vi "20220302-main.vi"() -> ()   [LabVIEW 2019]
uses:
  <vilib>/myRIO/Instrument Drivers/Utilities/Utilities.lvlib
  52/sub/servo state.ctl
  52/sub/state.ctl
  52/sub/route_name.ctl
  52/main data.ctl
  52/sub/vision/vision_board_ctl.ctl
  52/sub/block box.ctl
  52/sub/align position.ctl
  <vilib>/myRIO/Common/Instrument Driver Framework/myRIO v1.0/DIO/typedefs/DIO Channels Enum.ctl
  <vilib>/myRIO/Common/Instrument Driver Framework/myRIO v1.0/DIO/typedefs/DIO Channels List.ctl
  <vilib>/myRIO/Common/Instrument Driver Framework/Utilities/typedefs/Generic FPGA Reference.ctl
  <vilib>/myRIO/Common/Instrument Driver Framework/Utilities/typedefs/myRIO v1.0 Reference.ctl
  <vilib>/myRIO/Common/Instrument Driver Framework/Utilities/typedefs/Hardware Version Enum.ctl
  <vilib>/myRIO/Common/Instrument Driver Framework/Utilities/typedefs/myRIO Generic Hardware Reference.ctl
  <vilib>/myRIO/Instrument Drivers/Onboard IO/DIO/typedefs/DIO Reference.ctl
  <vilib>/myRIO/Instrument Drivers/Onboard IO/DIO/DIO.lvlib
  <vilib>/myRIO/Instrument Drivers/Onboard IO/DIO/vis/Write.vi
  <vilib>/userDefined/High Color/nirio_resource_hc.ctl
  <vilib>/myRIO/Common/Instrument Driver Framework/myRIO v1.0/DIO/vis/myRIO v1.1 Open DIO.vi
  <vilib>/myRIO/Instrument Drivers/Onboard IO/DIO/vis/myRIO DIO Open.xnode
  <vilib>/myRIO/Common/Instrument Driver Framework/Utilities/vis/Is FPGA Ref Available.vi
  <vilib>/myRIO/Express VI/Onboard Devices/LED/LED Express VI.xnode
  <vilib>/myRIO/Instrument Drivers/Onboard IO/DIO/vis/Read.vi
  <vilib>/myRIO/Express VI/Onboard Devices/Button/Button Express VI.xnode
  subVI/move control/move and align/move_cluster.ctl
  <vilib>/myRIO/Express VI/Onboard IO/DO/DO Express VI.xnode
panel:
  out "main.ctl":T1
  out "recycle?":bool
  in  "Error In":errorcluster
  out "error out":errorcluster
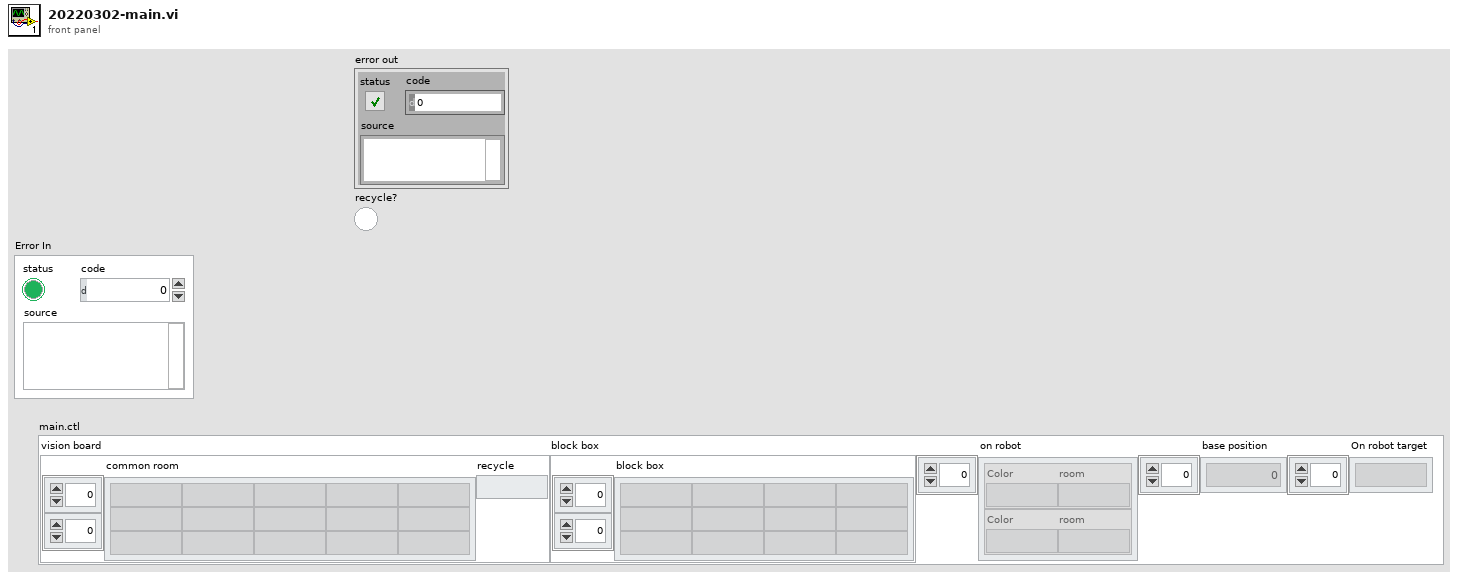
[diagram p1: front panel]
types:
  T1 = typedef "main data.ctl" = cluster{"vision board":T2, "block box":T3, "on robot ":cluster{"Color":string, "room":string}[], "base position":dbl[], "On robot target":string[]}
  T2 = typedef "vision_board_ctl.ctl" = cluster{"common room":string[][], "recycle":string}
  T3 = typedef "block box.ctl" = cluster{"block box":string[][]}
  T4 = typedef "state.ctl" = enum16{"vision", "catch", "recycle", "go home"}
  T5 = typedef "DIO.lvlib/DIO Reference.ctl" = cluster{"myRIO Reference":T6, "DIO Channels List":T10}
  T6 = typedef "myRIO Generic Hardware Reference.ctl" = cluster{"myRIO Model":T7, "myRIO Hardware Reference":T8}
  T7 = typedef "Hardware Version Enum.ctl" = enum16{"Unknown", "myRIO-1900", "myRIO-1950", "roboRIO", "NI ELVIS RIO CM", "ELVIS III"}
  T8 = typedef "myRIO v1.0 Reference.ctl" = cluster{"Generic FPGA Reference":T9, "Allow multiple opens":bool}
  T9 = typedef "Generic FPGA Reference.ctl" = refnum<k20>
  T10 = typedef "DIO Channels List.ctl" = T11[]
  T11 = typedef "DIO Channels Enum.ctl" = enum16{"Not Connected", "C/DIO0", "C/DIO1", "C/DIO2", "C/DIO3", "C/DIO4", "C/DIO5", "C/DIO6", "C/DIO7", "A/DIO0", "A/DIO1", "A/DIO2", "A/DIO3", "A/DIO4", "A/DIO5", "A/DIO6", "A/DIO7", "A/DIO8", "A/DIO9", "A/DIO10", "A/DIO11", "A/DIO12", "A/DIO13", "A/DIO14", "A/DIO15", "A/DIO16", "A/DIO17", "A/DIO18", "A/DIO19", "B/DIO0", "B/DIO1", "B/DIO2", "B/DIO3", "B/DIO4", "B/DIO5", "B/DIO6", "B/DIO7", "B/DIO8", "B/DIO9", "B/DIO10", "B/DIO11", "B/DIO12", "B/DIO13", "B/DIO14", "B/DIO15", "B/DIO16", "B/DIO17", "B/DIO18", "B/DIO19", "LED0", "LED1", "LED2", "LED3", "Button0", "DIO/DIO0", "DIO/DIO1", "DIO/DIO2", "DIO/DIO3", "DIO/DIO4", "DIO/DIO5", "DIO/DIO6", "DIO/DIO7", "DIO/DIO8", "DIO/DIO9", "SPI/CS0", "SPI/CS1", "SPI/CS2", "SPI/CS3", "LED RADIO (Green)", "LED RADIO (Red)", "LED COMM (Green)", "LED COMM (Red)", "LED MODE (Green)", "LED MODE (Red)"}
  T12 = typedef "nirio_resource_hc.ctl" = tag
  T13 = typedef "move_cluster.ctl" = cluster{"X":dbl, "Y":dbl, "degree":dbl, "speed":dbl}
  T14 = typedef "route_name.ctl" = enum16{"S-Vision", "Vision-R1", "Vision-R2", "Vision-R3", "Vision-R4", "Vision-R5", "R1-Vision", "R2-Vision", "R3-Vision", "R4-Vision", "R5-Vision", "Vision-box", "box-recycle", "recycle-box", "box-Vision", "Vision-S", "R2-R3"}
  T15 = typedef "servo state.ctl" = enum16{"catch", "cam-1", "put", "side", "center", "side-2", "put-2"}
  T16 = typedef "align position.ctl" = enum16{"S align", "vision align", "box align", "box to room align"}
  T17 = typedef "position cluster.ctl" = cluster{"X":dbl, "Y":dbl, "Angle":dbl}
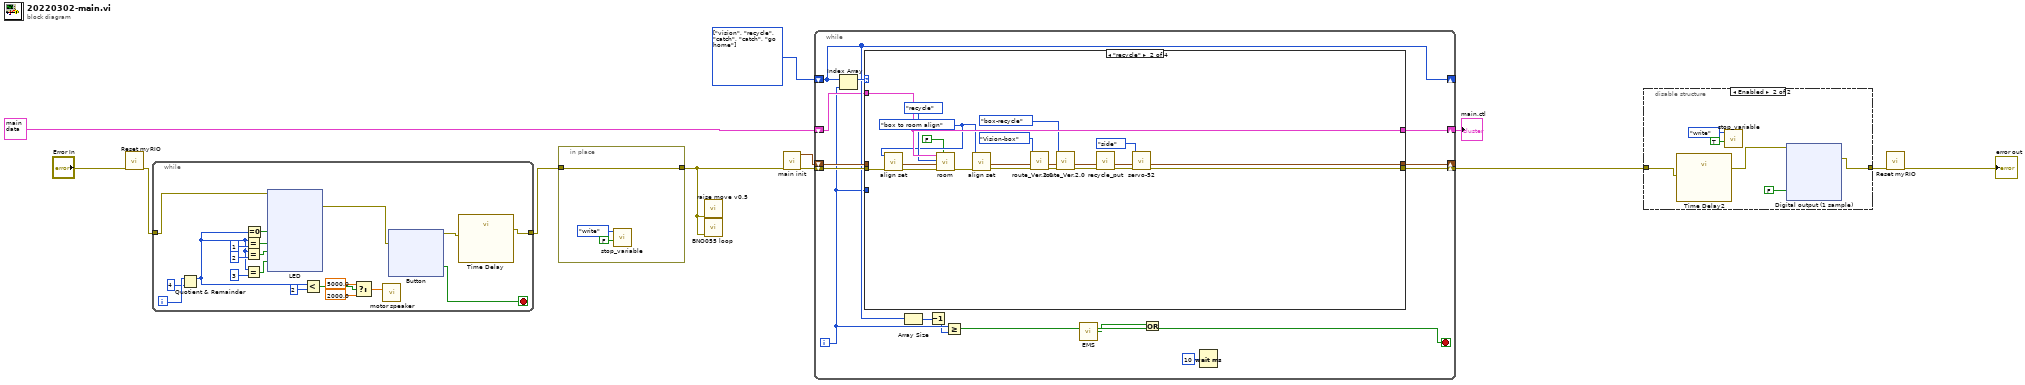
[diagram p0: block diagram]
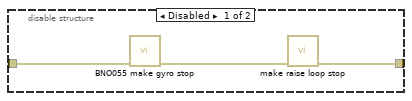
[diagram p2: hidden frame]
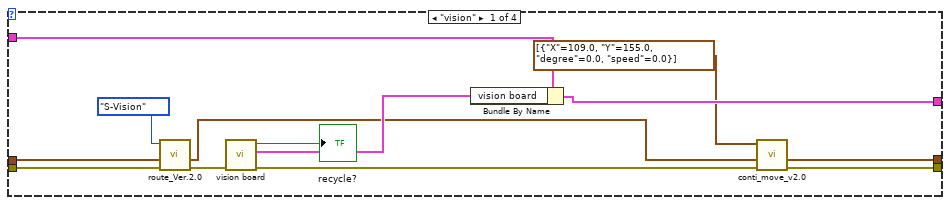
[diagram p3: hidden frame]
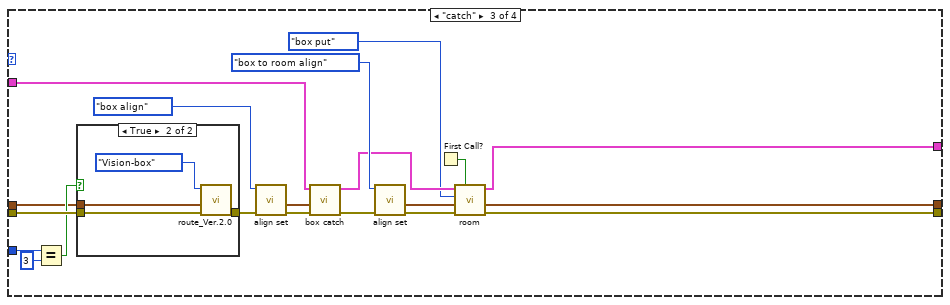
[diagram p4: hidden frame]
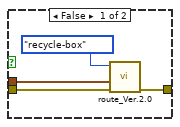
[diagram p5: hidden frame]
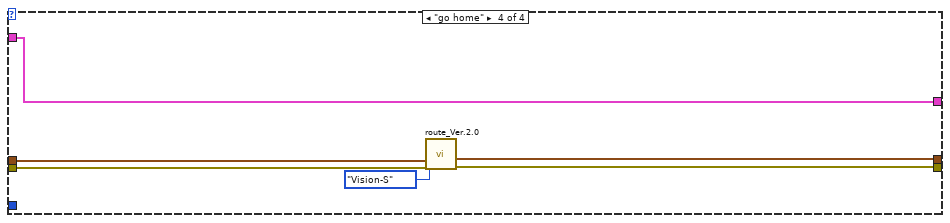
[diagram p6: hidden frame]
diagram:
  w9 = T4[] [enum."vision", enum."recycle", enum."catch", enum."catch", enum."go home"] items=["vision", "catch", "recycle", "go home"] ("Array")
  n1 = call <vilib>:"Reset myRIO.vi"("error in (no error)"="Error In") -> ("error out"=w2:errorcluster)  [unwired: 10 in]
  n2 = while {
    tunnel: w2 -> [w23]
    tunnel: [w20] -> w1
    i -> [w32]
    stop <- w21 stop-if-true
    n3 = Quotient & Remainder(x=w32, y=4) -> (x-y*floor(x/y)=w18:i32)  [unwired: 1 out]
    n4 = Equal?(x=w18, y=1) -> (x = y?=w29:bool)
    n5 = Equal?(x=w18, y=2) -> (x = y?=w26:bool)
    n6 = Equal?(x=w18, y=3) -> (x = y?=w25:bool)
    n7 = Equal To 0?(x=w18) -> (x = 0?=w30:bool)
    n8 = xnode "LED"("LED0"=w30, "LED1"=w29, "LED2"=w26, "LED3"=w25, "error in (no error)"=w23) -> ("error out"=w22:errorcluster)
    n9 = Less?(x=w18, y=2) -> (x < y?=w15:bool)
    n10 = Select(t=5000.0, s=w15, f=2000.0) -> (s? t:f=w16:dbl)
    n11 = call "motor speaker.vi"("Vertical Pointer Slide"=w16) -> ()  [unwired: 11 in]
    n12 = xnode "Button"("error in (no error)"=w22) -> ("Value"=w21:bool, "error out"=w19:errorcluster)
    n13 = call "Time Delay"("error in (no error)"=w19) -> ("error out"=w20:errorcluster)  [unwired: 10 in]
  }
  n14 = in-place {
    in-place-border: [w108] -> w3
    in-place-border: w1 -> [w108]
    n15 = call "stop_variable.vi"("Write"=FALSE, "Enum"=enum16{"read", "write"}."write") -> ()  [unwired: 9 in, 1 out]
  }
  n16 = call "raise move v0.5.vi"("error in (no error)"=w3) -> ()  [unwired: 10 in, 1 out]
  n17 = call "BNO055 loop.vi"("error in (no error)"=w3) -> ()  [unwired: 11 in]
  n18 = call "main init.vi"("error in (no error)"=w3) -> ("error out"=w12:errorcluster, "position out"=w11:cluster{"x":dbl, "y":dbl, "degree":dbl})  [unwired: 9 in]
  n19 = while {
    shift-right: [w118] -> _
    shift-left: w9 -> [w118]
    shift-right: [w121] -> w10
    shift-left: w12 -> [w123]
    shift-right: [w119] -> _
    shift-left: w11 -> [w122]
    shift-right: [w114] -> w6
    shift-left: T1 {"vision board"={"common room"=[["", "green", "", "blue", ""], ["", "red", "", "black", ""], ["", "", "", "", ""]], "recycle"="R1"}, "block box"={"block box"=[]}, "on robot "=[{"Color"="", "room"=""}, {"Color"="", "room"=""}], "base position"=[], "On robot target"=[]} -> [w115]
    i -> [w111]
    stop <- w113 stop-if-true
    n20 = Index Array(array=w118, index=w111) -> (element=w120:T4)
    n21 = case shown="\"recycle\"" w120 {
      tunnel: w123 -> [w136 w138 w171 w187]
      tunnel: w122 -> [w135 _ w165 w186]
      tunnel: [w128 w142 w161 w188] -> w121
      tunnel: [w127 w145 w160 w189] -> w119
      tunnel: w115 -> [w132 w156 w172 w185]
      tunnel: [w131 w156 w159 w185] -> w114
      tunnel: w111 -> [_ _ w168 _]
      frame "vision" {
        n22 = call "route_Ver.2.0.vi"("error in (no error)"=w136, "Position"=w135, 11:route_name."S-Vision") -> ("error out"=w133:errorcluster, "Position out"=w126:T17)  [unwired: 7 in]
        n23 = call "vision board.vi"("error in (no error)"=w133) -> ("error out"=w124:errorcluster, "vision board"=w130:T2, "recycle?"=→"recycle?":bool)  [unwired: 8 in]
        n24 = Bundle By Name(cluster=w132, "vision board"=w130) -> (w131:T1)
        n25 = call "conti_move_v2.0.vi"("error in (no error)"=w124, "Position"=w126, "route"=T13[] [{"X"=109.0, "Y"=155.0, "degree"=0.0, "speed"=0.0}]) -> ("error out"=w128:errorcluster, "Position out"=w127:T17)  [unwired: 7 in]
      }
      frame "recycle" {
        w141 = align_position."box to room align" ("align position")
        n26 = call "align set.vi"("error in (no error)"=w138, "align position"=w141) -> ("error out"=w139:errorcluster, "position out"=w140:cluster{"X":dbl, "y":dbl, "degree":dbl})  [unwired: 8 in]
        n27 = call "room.vi"("conti R3?"=FALSE, "error in (no error)"=w139, "Position"=w140, "Enum"=enum16{"recycle", "box put"}."recycle", "main.ctl"=w156) -> ("error out"=w150:errorcluster)  [unwired: 4 in, 2 out]
        n28 = call "align set.vi"("error in (no error)"=w150, "align position"=w141) -> ("error out"=w149:errorcluster, "position out"=w148:cluster{"X":dbl, "y":dbl, "degree":dbl})  [unwired: 8 in]
        n29 = call "route_Ver.2.0.vi"("error in (no error)"=w149, "Position"=w148, 11:route_name."Vision-box") -> ("error out"=w153:errorcluster, "Position out"=w152:T17)  [unwired: 7 in]
        n30 = call "route_Ver.2.0.vi"("error in (no error)"=w153, "Position"=w152, 11:route_name."box-recycle") -> ("error out"=w146:errorcluster, "Position out"=w147:T17)  [unwired: 7 in]
        n31 = call "recycle_put.vi"("Error In"=w146, "Position In"=w147) -> ("Error Out"=w144:errorcluster, "Position out"=w145:T17)  [unwired: 8 in]
        n32 = call "servo-52.vi"("error in (no error)"=w144, "Enum"=servo_state."side") -> ("error out"=w142:errorcluster)  [unwired: 9 in]
      }
      frame "catch" {
        n33 = Equal?(x=w168, y=3) -> (x = y?=w166:bool)
        n34 = case shown="True" w166 {
          tunnel: [w180 w184] -> w176
          tunnel: w171 -> [w179 w182]
          tunnel: w165 -> [w178 w181]
          frame False {
            n35 = call "route_Ver.2.0.vi"("error in (no error)"=w179, "Position"=w178, 11:route_name."recycle-box") -> ("error out"=w180:errorcluster)  [unwired: 7 in, 1 out]
          }
          frame True {
            n36 = call "route_Ver.2.0.vi"("error in (no error)"=w182, "Position"=w181, 11:route_name."Vision-box") -> ("error out"=w184:errorcluster)  [unwired: 7 in, 1 out]
          }
        }
        n37 = call "align set.vi"("error in (no error)"=w176, "align position"=align_position."box align") -> ("error out"=w174:errorcluster, "position out"=w173:cluster{"X":dbl, "y":dbl, "degree":dbl})  [unwired: 8 in]
        n38 = call "box catch.vi"("Error In"=w174, "Position in"=w173, "main.ctl"=w172) -> ("Error Out"=w170:errorcluster, "main.ctl 2"=w164:T1)  [unwired: 6 in, 1 out]
        n39 = call "align set.vi"("error in (no error)"=w170, "align position"=align_position."box to room align") -> ("error out"=w162:errorcluster, "position out"=w163:cluster{"X":dbl, "y":dbl, "degree":dbl})  [unwired: 8 in]
        n40 = First Call?() -> (First Call?: T/F=w157:bool)
        n41 = call "room.vi"("conti R3?"=w157, "error in (no error)"=w162, "Position"=w163, "Enum"=enum16{"recycle", "box put"}."box put", "main.ctl"=w164) -> ("error out"=w161:errorcluster, "Position out"=w160:T17, "main.ctl 2"=w159:T1)  [unwired: 4 in]
      }
      frame "go home" {
        n42 = call "route_Ver.2.0.vi"("error in (no error)"=w187, "Position"=w186, 11:route_name."Vision-S") -> ("error out"=w188:errorcluster, "Position out"=w189:T17)  [unwired: 7 in]
      }
    }
    n43 = Array Size(array=w118) -> (size(s)=w117:i32)
    n44 = Decrement(x=w117) -> (x-1=w110:i32)
    n45 = Greater Or Equal?(x=w111, y=w110) -> (x >= y?=w116:bool)
    n46 = call "EMS.vi"() -> ("A/DIO4 (Pin 19)"=w112:bool)
    n47 = Or(x=w112, y=w116) -> (x .or. y?=w113:bool)
    n48 = Wait (ms)(milliseconds to wait=u32 10) -> ()  [unwired: 1 out]
  }
  "main.ctl" <- w6
  n49 = disable-structure shown="Enabled" {
    disable-tunnel: w10 -> [w193 w196]
    disable-tunnel: [w192 w194] -> w4
    frame Disabled {
      n50 = call "BNO055 make gyro stop .vi"("error in (no error)"=w193) -> ("error out"=w191:errorcluster)  [unwired: 10 in]
      n51 = call "make raise loop stop.vi"("error in (no error)"=w191) -> ("error out"=w192:errorcluster)  [unwired: 10 in]
    }
    frame Enabled {
      n52 = call "Time Delay2"("error in (no error)"=w196) -> ("error out"=w195:errorcluster)  [unwired: 10 in]
      n53 = call "stop_variable.vi"("Write"=TRUE, "Enum"=enum16{"read", "write"}."write") -> ()  [unwired: 9 in, 1 out]
      n54 = xnode "Digital output (1 sample)"("C/DIO1 (DIO1)"=FALSE, "error in (no error)"=w195) -> ("error out"=w194:errorcluster)
    }
  }
  n55 = call <vilib>:"Reset myRIO.vi"("error in (no error)"=w4) -> ("error out"=→"error out":errorcluster)  [unwired: 10 in]
